vi "DCPower.vi"() -> ()   [LabVIEW 2022 SP3]
uses:
  <vilib>/DAQmx/read.llb/DAQmx Read (Digital Bool 1Line 1Point).vi
  <vilib>/DAQmx/create/channels.llb/DAQmx Create Channel (DI-Digital Input).vi
  <vilib>/DAQmx/miscellaneous.llb/DAQmx Fill In Error Info.vi
panel:
  out "error out":errorcluster
  out "connected":bool
  in  "VISA resource name":refnum<visa-resource-name>
  out "Boolean":bool
  in  "Numeric 3":dbl
  in  "stop":bool
  in  "lines":tag
  in  "Connect":bool
  in  "Numeric":dbl
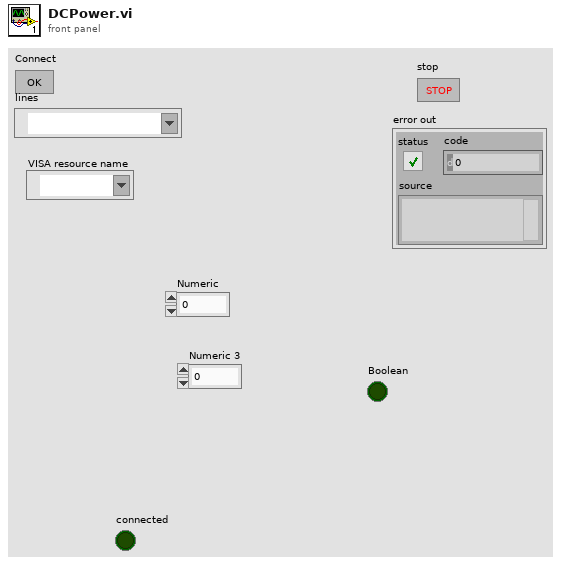
[diagram p1: front panel]
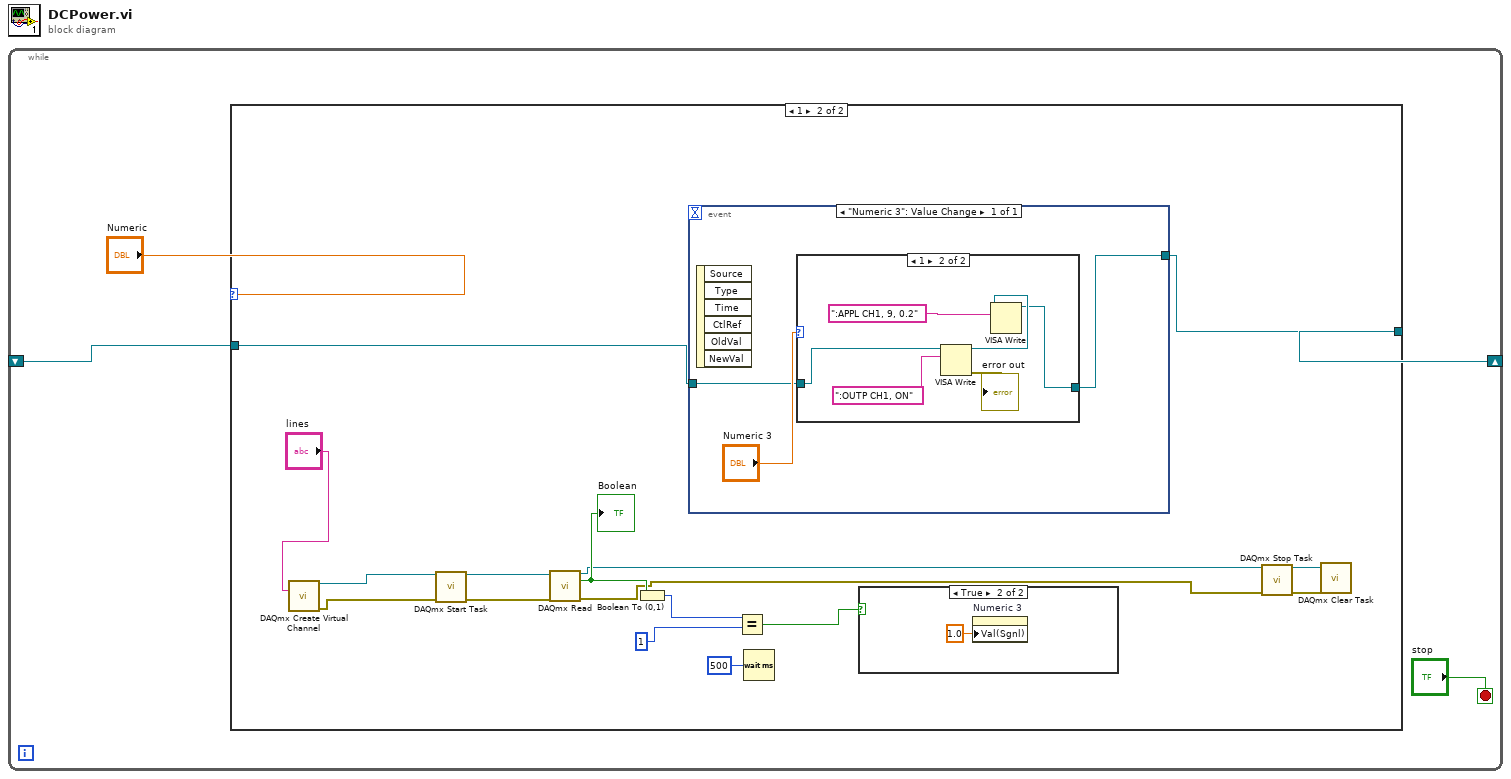
[diagram p0: block diagram]
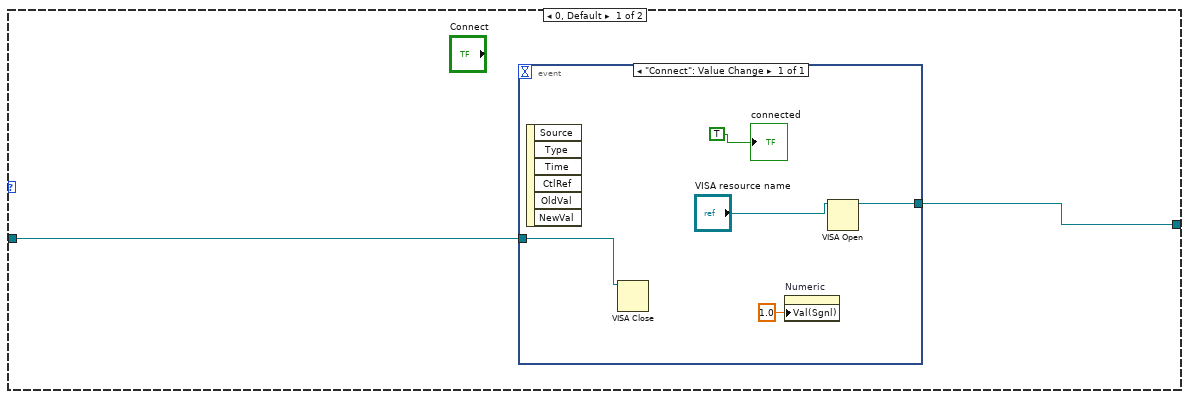
[diagram p2: hidden frame]
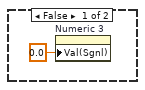
[diagram p3: hidden frame]
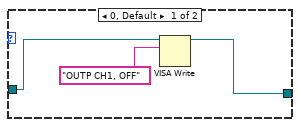
[diagram p4: hidden frame]
diagram:
  n1 = while {
    shift-right: [w4] -> _
    shift-left: _ -> [w2]
    stop <- "stop" stop-if-true
    n2 = case shown="1" "Numeric" {
      tunnel: [w5 w27] -> w4
      tunnel: w2 -> [w6 w26]
      frame 0, Default {
        n3 = event shown="[0] \"Connect\": Value Change" {
          selector: _ -> [_]
          dyn-events: _ -> [_]
          timeout: _ -> [_]
          tunnel: w6 -> [w11]
          tunnel: [w9] -> w5
          event "Connect": Value Change {
            n4 = event-data() -> ()  [unwired: 1 in, 6 out]
            n5 = VISA Close(VISA resource name=w11) -> ()  [unwired: 1 in, 1 out]
            n6 = property on="Numeric" class="DigNum (strict)"("Val(Sgnl)"=1.0 ("Value (Signaling)")) -> ()  [unwired: 2 in, 2 out]
            n7 = VISA Open(VISA resource name="VISA resource name") -> (VISA resource name=w9:refnum<visa-resource-name>)  [unwired: 4 in, 1 out]
            "connected" <- TRUE
          }
        }
      }
      frame 1 {
        n8 = call-poly <vilib>:"DAQmx Create Virtual Channel.vi"("lines"="lines") -> ("task out"=w19:refnum<k21>, "error out"=w18:errorcluster)  [unwired: 13 in]
        n9 = call <vilib>:"DAQmx Start Task.vi"("task/channels in"=w19, "error in"=w18) -> ("task out"=w21:refnum<k21>, "error out"=w20:errorcluster)  [unwired: 12 in]
        n10 = call-poly <vilib>:"DAQmx Read.vi"("task/channels in"=w21, "error in"=w20) -> ("task out"=w16:refnum<k21>, "data"=w22:bool, "error out"=w15:errorcluster)  [unwired: 11 in]
        "Boolean" <- w22
        n11 = Boolean To (0,1)(Boolean=w22) -> (0, 1=w24:i16)
        n12 = event shown="[0] \"Numeric 3\": Value Change" {
          selector: _ -> [_]
          dyn-events: _ -> [_]
          timeout: _ -> [_]
          tunnel: [w32] -> w27
          tunnel: w26 -> [w30]
          event "Numeric 3": Value Change {
            n13 = event-data() -> ()  [unwired: 1 in, 6 out]
            n14 = case shown="1" "Numeric 3" {
              tunnel: [w34 w38] -> w32
              tunnel: w30 -> [w33 w37]
              frame 0, Default {
                n15 = VISA Write(VISA resource name=w33, write buffer="OUTP CH1, OFF") -> (VISA resource name out=w34:refnum<visa-resource-name>)  [unwired: 1 in, 2 out]
              }
              frame 1 {
                n16 = VISA Write(VISA resource name=w37, write buffer=":OUTP CH1, ON") -> (VISA resource name out=w39:refnum<visa-resource-name>, error out=→"error out":errorcluster)  [unwired: 1 in, 1 out]
                n17 = VISA Write(VISA resource name=w39, write buffer=":APPL CH1, 9, 0.2") -> (VISA resource name out=w38:refnum<visa-resource-name>)  [unwired: 1 in, 2 out]
              }
            }
          }
        }
        n18 = Equal?(x=w24, y=1) -> (x = y?=w25:bool)
        n19 = Wait (ms)(milliseconds to wait=u32 500) -> ()  [unwired: 1 out]
        n20 = case shown="True" w25 {
          frame False {
            n21 = property on="Numeric 3" class="DigNum (strict)"("Val(Sgnl)"=0.0 ("Value (Signaling)")) -> ()  [unwired: 2 in, 2 out]
          }
          frame True {
            n22 = property on="Numeric 3" class="DigNum (strict)"("Val(Sgnl)"=1.0 ("Value (Signaling)")) -> ()  [unwired: 2 in, 2 out]
          }
        }
        n23 = call <vilib>:"DAQmx Stop Task.vi"("task/channels in"=w16, "error in"=w15) -> ("task out"=w14:refnum<k21>, "error out"=w13:errorcluster)  [unwired: 12 in]
        n24 = call <vilib>:"DAQmx Clear Task.vi"("task in"=w14, "error in"=w13) -> ()  [unwired: 13 in, 1 out]
      }
    }
  }
